vi "Read User Data.vi"(11 "RT Data in":T1 {"Block Data Refs"."Data Reference" format="%.0x"}) -> (3 "RT Data out":T1 {"Block Data Refs"."Data Reference" format="%.0x"})   [LabVIEW 2011, in "Sensor Simulation Custom Device.lvlib"]
uses:
  Sensor Simulation Custom Device.lvlib
  TypeDefs/SensorStateVariables.ctl
  <userlib>/_FPGA Interface Advanced Tools/FPGA Interface Base/FPGA Interface Base.lvclass
  TypeDefs/4 Wire xVDT Parameters.ctl
  TypeDefs/5 Wire xVDT Parameters.ctl
  TypeDefs/Resolver Parameters.ctl
  <vilib>/NI Veristand/Custom Device API/Block Data Reference.ctl
  <vilib>/NI Veristand/Custom Device API/Data Reference.ctl
  <vilib>/NI Veristand/Custom Device API/Global Data Refs.vi
  <vilib>/NI Veristand/Custom Device API/Custom Device API.lvlib
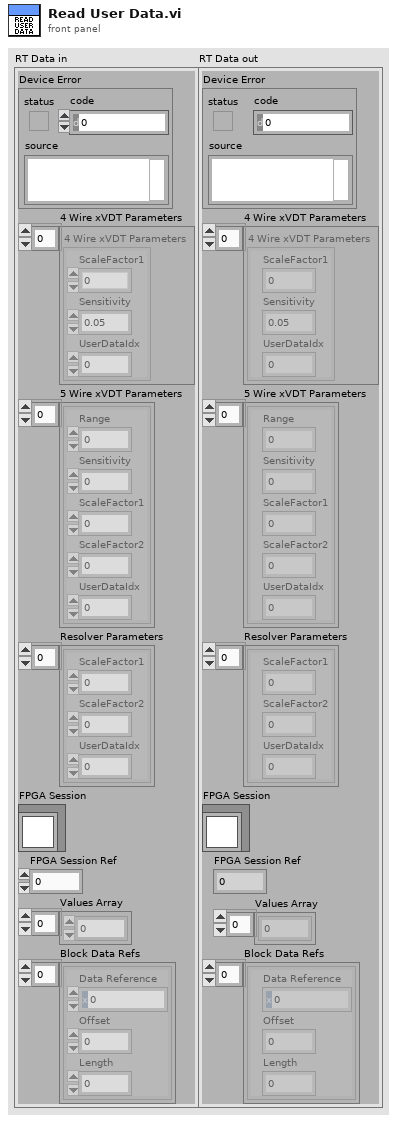
[diagram p1: front panel]
types:
  T1 = typedef "Sensor Simulation Custom Device.lvlib/SensorStateVariables.ctl" = cluster{"Device Error":errorcluster, "4 Wire xVDT Parameters ":T2[], "5 Wire xVDT Parameters":T3[], "Resolver Parameters":T4[], "FPGA Session":refnum<class "FPGA Interface Base.lvclass">, "FPGA Session Ref":u32, "Values Array":dbl[], "Block Data Refs":T5[]}
  T2 = typedef "Sensor Simulation Custom Device.lvlib/4 Wire xVDT Parameters.ctl" = cluster{"ScaleFactor1":u32, "Sensitivity":dbl, "UserDataIdx":i32}
  T3 = typedef "Sensor Simulation Custom Device.lvlib/5 Wire xVDT Parameters.ctl" = cluster{"Range":dbl, "Sensitivity":dbl, "ScaleFactor1":u32, "ScaleFactor2":u32, "UserDataIdx":i32}
  T4 = typedef "Sensor Simulation Custom Device.lvlib/Resolver Parameters.ctl" = cluster{"ScaleFactor1":u32, "ScaleFactor2":u32, "UserDataIdx":i32}
  T5 = typedef "Custom Device API.lvlib/Block Data Reference.ctl" = cluster{"Data Reference":T6, "Offset":i32, "Length":i32}
  T6 = typedef "Custom Device API.lvlib/Data Reference.ctl" = i32
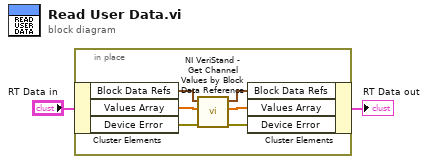
[diagram p0: block diagram]
diagram:
  n1 = in-place {
    n2 = in-place-cluster #1("RT Data in") -> ("Block Data Refs"=w6:T5[], "Values Array"=w7:dbl[], "Device Error"=w8:errorcluster)
    n3 = call <vilib>:"NI VeriStand - Get Channel Values by Block Data Reference.vi"("error in (no error)"=w8, "Values Array in"=w7, "Block Data Ref"=w6) -> ("error out"=w3:errorcluster, "Values Array out"=w4:dbl[], "Block Data Ref dup"=w5:T5[])  [unwired: 6 in]
    n4 = in-place-cluster #1("Block Data Refs"=w5, "Values Array"=w4, "Device Error"=w3) -> (→"RT Data out":T1)
  }
